vi "ADXL345 I2C Open.vi"(8 "error in (no error)":errorcluster, 9 "Range":T3 items=["+/- 2 g", "+/- 4 g", "+/- 8 g", "+/- 16 g"], 11 "DIO Module (Module 1)":T2=enum."Digital Module 2") -> (0 "error out":errorcluster, 3 "I2CDevRef":T1 {"Device Address" format="%.0x"})   [LabVIEW 2012]
uses:
  <vilib>/Rock Robotics/SystemInterfaces/Typedef/FPGA_TypedefDigitalModule.ctl
  ADXL345 I2C Range.ctl
  <vilib>/Rock Robotics/WPI/I2C/WPI_I2CDevRef.ctl
  <vilib>/Rock Robotics/SystemInterfaces/NetworkCommunication/NetComm_UsageReport_ResourceType.ctl
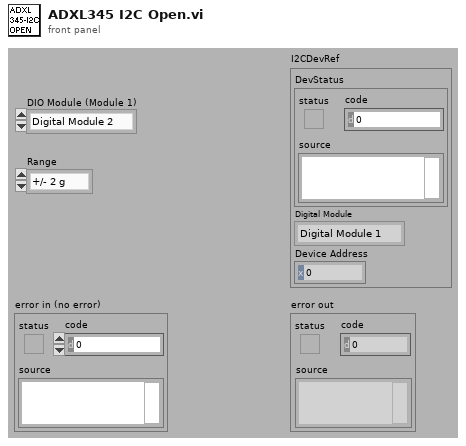
[diagram p1: front panel]
types:
  T1 = typedef "WPI_I2CDevRef.ctl" = cluster{"DevStatus":errorcluster, "Digital Module":T2, "Device Address":u8}
  T2 = typedef "FPGA_TypedefDigitalModule.ctl" = enum16{"Digital Module 1", "Digital Module 2"}
  T3 = typedef "ADXL345 I2C Range.ctl" = u8
  T4 = typedef "NetComm_UsageReport_ResourceType.ctl" = enum8{"Controller", "Module", "Language", "CANPlugin", "Accelerometer", "ADXL345", "AnalogChannel", "AnalogTrigger", "AnalogTriggerOutput", "CANJaguar", "Compressor", "Counter", "Dashboard", "DigitalInput", "DigitalOutput", "DriverStationCIO", "DriverStationEIO", "DriverStationLCD", "Encoder", "GearTooth", "Gyro", "I2C", "Framework", "Jaguar", "Joystick", "Kinect", "KinectStick", "PIDController", "Preferences", "PWM", "Relay", "RobotDrive", "SerialPort", "Servo", "Solenoid", "SPI", "Task", "Ultrasonic", "Victor", "Button", "Command", "AxisCamera", "PCVideoServer", "SmartDashboard", "Talon", "HiTechnicColorSensor", "HiTechnicAccel", "HiTechnicCompass", "SRF08"}
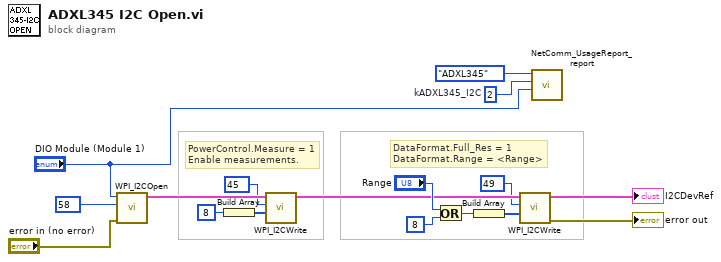
[diagram p0: block diagram]
diagram:
  w2 = u8 2  # kADXL345_I2C
  # "DataFormat.Full_Res = 1\nDataFormat.Range = <Range>"
  # "PowerControl.Measure = 1\nEnable measurements."
  n1 = call <vilib>:"WPI_I2COpen.vi"("error in"="error in (no error)", "Device Address"=u8 58 ("Data To Send"), "Digital Module (Module 1)"="DIO Module (Module 1)") -> ("I2CDevRef"=w11:T1)  [unwired: 8 out]
  n2 = Build Array(u8 8 ("Data To Send")) -> (w8:u8[])
  n3 = call <vilib>:"WPI_I2CWrite.vi"("I2CDataToSend"=w8, "I2CRegister"=u8 45 ("Data To Send"), "I2CDevRef"=w11) -> ("I2CDevRef"=w14:T1)  [unwired: 2 in, 6 out]
  n4 = Or(x="Range", y=u8 8 ("Data To Send")) -> (x .or. y?=w7:T3)
  n5 = Build Array(w7) -> (w6:T3[])
  n6 = call <vilib>:"WPI_I2CWrite.vi"("I2CDataToSend"=w6, "I2CRegister"=u8 49 ("Data To Send"), "I2CDevRef"=w14) -> ("error out"=→"error out":errorcluster, "I2CDevRef"=→"I2CDevRef":T1)  [unwired: 2 in, 5 out]
  n7 = call <vilib>:"NetComm_UsageReport_report.vi"("Context"="DIO Module (Module 1)", "Instance Number"=w2, "Resource Type"=NetComm_UsageReport_ResourceType."ADXL345") -> ()  [unwired: 9 in]
